vi "TreeNode Put Timestamped Segment.vi"(0 "TreeNode DVR in":refnum<data-value>, 5 "Segment Data":refnum<data-value>, 7 "Timestamps":refnum<data-value>, 11 "error in (no error)":errorcluster) -> (4 "TreeNode DVR out":refnum<data-value>, 15 "error out":errorcluster)   [LabVIEW 2015, in "MDSplus.lvlib"]
doc: "Write a single row of timestamped data."
uses:
  <vilib>/MDSplus/Library/MDSplus.lvlib
  <vilib>/MDSplus/Classes/Data_Class/TreeNode_Class/TreeNode.lvclass
  <vilib>/MDSplus/Classes/Data_Class/Data.lvclass
  <vilib>/MDSplus/Classes/Data_Class/Array_Class/Int64Array_Class/Int64Array.lvclass
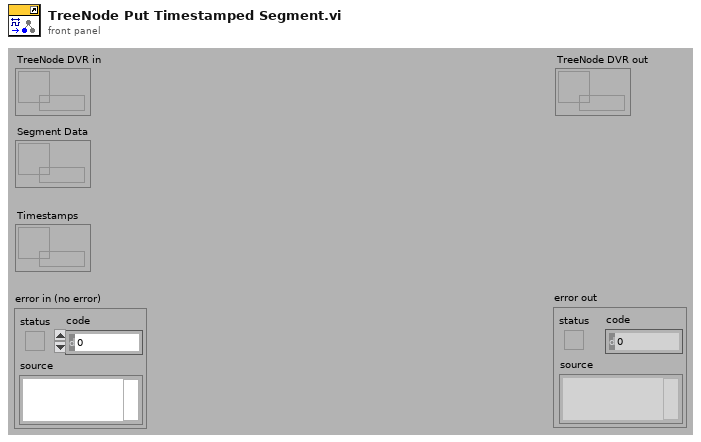
[diagram p1: front panel]
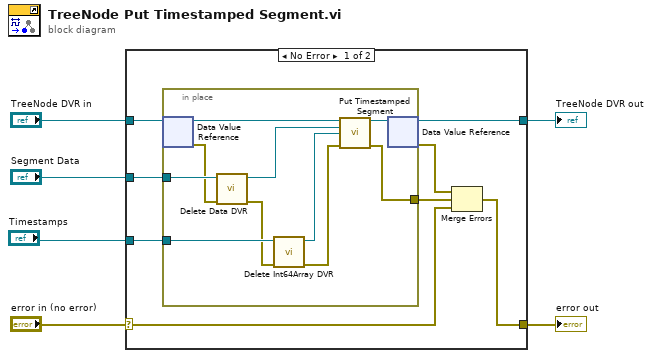
[diagram p0: block diagram]
diagram:
  n1 = case shown="No Error" "error in (no error)" {
    selector: "error in (no error)" -> [w13 w25]
    tunnel: "TreeNode DVR in" -> [w14 w26]
    tunnel: [w10 w25] -> w6
    tunnel: [w11 w26] -> w3
    tunnel: "Segment Data" -> [w8 _]
    tunnel: "Timestamps" -> [w7 _]
    frame No Error {
      n2 = in-place {
        in-place-border: [w15] -> w9
        in-place-border: w8 -> [w24]
        in-place-border: w7 -> [w22]
        n3 = in-place-dvr #1(w14) -> (w20:refnum<class "TreeNode.lvclass">, w23:errorcluster)
        n4 = call <vilib>:"Delete Data DVR.vi"("error in (no error)"=w23, "Data DVR in"=w24) -> ("error out"=w21:errorcluster, "Data out"=w18:refnum<class "Data.lvclass">)  [unwired: 8 in]
        n5 = call <vilib>:"Delete Int64Array DVR.vi"("error in (no error)"=w21, "Int64Array DVR in"=w22) -> ("error out"=w17:errorcluster, "Int64Array out"=w16:refnum<class "Int64Array.lvclass">)  [unwired: 8 in]
        n6 = call-dynamic "Put Timestamped Segment.vi"("TreeNode in"=w20, "Segment data"=w18, "Timestamps"=w16, "error in (no error)"=w17) -> ("TreeNode out"=w19:refnum<class "TreeNode.lvclass">, "error out"=w15:errorcluster)  [unwired: 10 in]
        n7 = in-place-dvr #1(w19) -> (w11:refnum<data-value>, w12:errorcluster)
      }
      n8 = Merge Errors(w12, w9, w13) -> (w10:errorcluster)
    }
    frame Error {
    }
  }
  "error out" <- w6
  "TreeNode DVR out" <- w3
